vi "Setting a new Protocol.vi"(8 "error in (no error)":errorcluster, 11 "instrument addon refnum in":T1 format="%.0x") -> (0 "error out":errorcluster, 3 "instrument addon refnum out":T1=18446744073709551615 format="%.0x")   [LabVIEW 2018]
uses:
  <vilib>/NI Veristand/Custom Device API/Custom Device Item Ref.ctl
  <vilib>/addons/VeriStand Custom Device Scripting APIs/Instrument Addon/Libraries Directory/Protocols.lvlibp/TCP/TCP Settings.ctl
  <vilib>/addons/VeriStand Custom Device Scripting APIs/Instrument Addon/API/Custom Device/TCP Factory.vi
  <vilib>/addons/VeriStand Custom Device Scripting APIs/Instrument Addon/API/Instrument Addon Scripting API.lvlib
  <vilib>/addons/VeriStand Custom Device Scripting APIs/Instrument Addon/Libraries Directory/Protocols.lvlibp/TCP/TCP.lvclass
  <vilib>/NI Veristand/Custom Device API/Custom Device API.lvlib
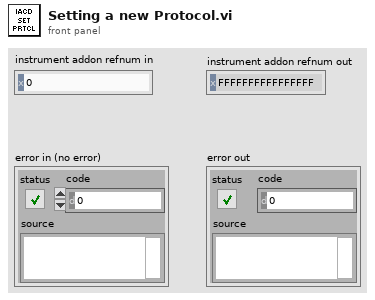
[diagram p1: front panel]
types:
  T1 = typedef "Custom Device API.lvlib/Custom Device Item Ref.ctl" = u64
  T2 = typedef "Protocols.lvlibp/TCP.lvclass/TCP Settings.ctl" = cluster{"IP Address":string, "Port":u16}
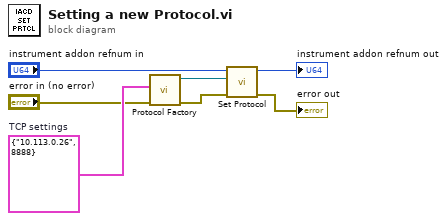
[diagram p0: block diagram]
diagram:
  w5 = T2 {"IP Address"="10.113.0.26", "Port"=8888}  # TCP settings
  n1 = call-poly <vilib>:"Protocol Factory.vi"("error in (no error)"="error in (no error)", "settings"=w5) -> ("error out"=w3:errorcluster, "protocol out"=w6:refnum<class "Protocol Parent.lvclass">)  [unwired: 8 in]
  n2 = call <vilib>:"Set Protocol.vi"("error in (no error)"=w3, "protocol"=w6, "instrument addon refnum in"="instrument addon refnum in") -> ("error out"=→"error out":errorcluster, "instrument addon refnum out"=→"instrument addon refnum out":T1)  [unwired: 7 in]
